vi "Scattered 2D Interpolation.vi"() -> ()   [LabVIEW 2023]
doc: "Illustrates how to use the Interpolate 2D Scattered VI to perform interpolation on scattered and grid data."
uses:
  <vilib>/Math Plots/3D Math Plots/3D Scatter/3D Scatter XCtrl/3D Scatter.xctl
  <vilib>/Math Plots/3D Math Plots/3D Surface/3D Surface XCtrl/3D Surface.xctl
  <vilib>/Analysis/1siggen.llb/Ramp Pattern by Samples.vi
  <vilib>/gmath/interp.llb/Create Mesh Grid (2D) (x,y arrays).vi
  <vilib>/Math Plots/3D Math Plots/3D Scatter/3D Scatter Datatype/Public/Plot Helper (Vector).vi
  <vilib>/gmath/interp.llb/Interpolate 2D Scattered (2D).vi
  <vilib>/Math Plots/3D Math Plots/3D Surface/3D Surface Datatype/Public/Plot Helper (Matrix).vi
  <vilib>/Analysis/NI_AALBase.lvlib
  <vilib>/gmath/NI_AAL_Interpolation.lvlib
  <vilib>/gmath/NI_Gmath.lvlib
  <vilib>/Math Plots/3D Math Plots/3D Scatter/3D Scatter Datatype/3D Scatter Datatype.lvclass
  <vilib>/Math Plots/3D Math Plots/3D Surface/3D Surface Datatype/3D Surface Datatype.lvclass
panel:
  out "Interpolation":refnum<class "3D Plot Datatype.lvclass">[](xcontrol)
  out "Raw Data":refnum<class "3D Plot Datatype.lvclass">[](xcontrol)
  in  "Data":u16(ring) items=["Scattered Data", "Grid Data"]
  in  "Method":i32(ring)=1 items=["nearest", "linear", "cubic", "biharmonic spline "]
  # "Overview: Illustrates how to use the Interpolate 2D Scattered VI to perform interpolation on scattered and grid data.\nRequirements: LabVIEW Full Development System\nInstructions: \n1. Use the Data option to choose between scattered or grid data.\n2. Use the Method option to choose the interpolation method.\n3. Run the VI.\n4. Observe the difference in input data types and interpolation methods on the Raw Data and Interpolation graphs."
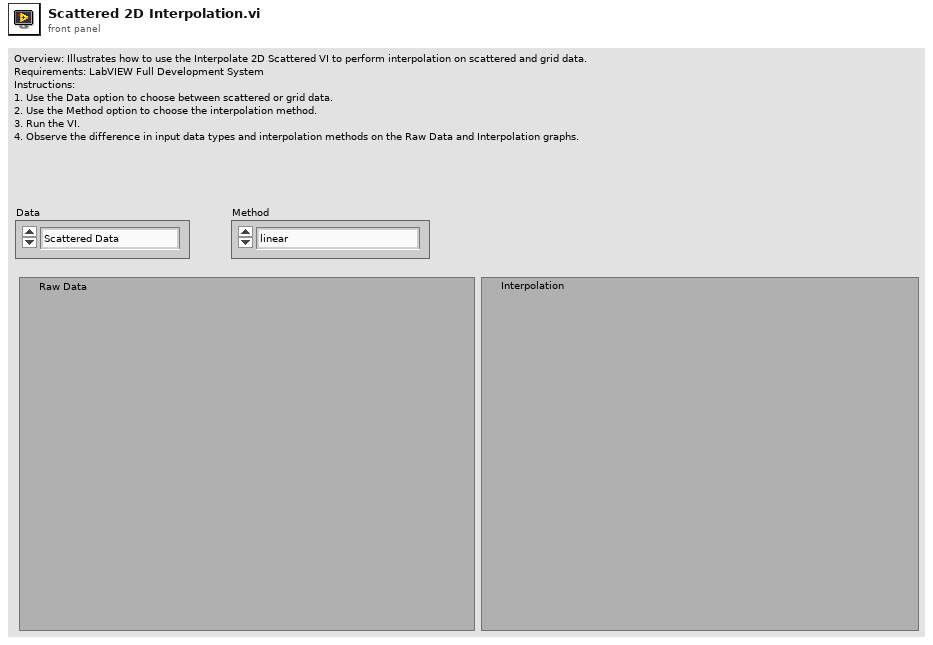
[diagram p1: front panel]
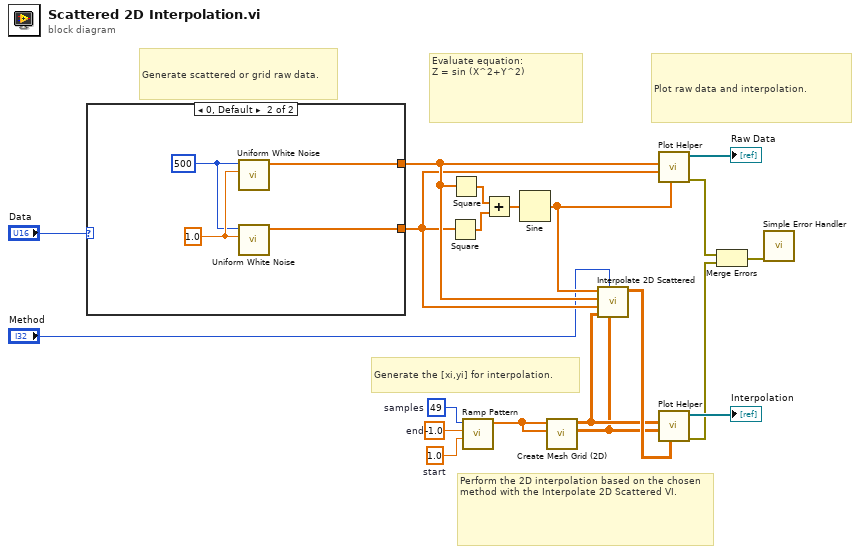
[diagram p0: block diagram]
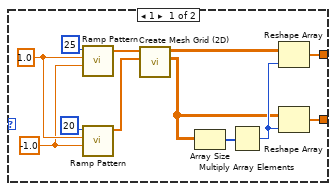
[diagram p2: hidden frame]
diagram:
  w13 = 1.0  # start
  w15 = 49  # samples
  w16 = -1.0  # end
  # "Generate the [xi,yi] for interpolation."
  # "Generate scattered or grid raw data."
  # "Perform the 2D interpolation based on the chosen method with the Interpolate 2D Scattered VI."
  # "Plot raw data and interpolation."
  # "Evaluate equation:\nZ = sin (X^2+Y^2)"
  n1 = case shown="0, Default" "Data" {
    tunnel: [w23 w33] -> w11
    tunnel: [w22 w34] -> w10
    frame 1 {
      w21 = -1.0 ("start")
      w31 = 1.0
      n2 = call-poly <vilib>:"Ramp Pattern.vi"("start"=w21, "end"=w31, "samples"=25) -> ("Ramp Pattern"=w30:dbl[])  [unwired: 7 in, 1 out]
      n3 = call-poly <vilib>:"Ramp Pattern.vi"("start"=w21, "end"=w31, "samples"=20) -> ("Ramp Pattern"=w29:dbl[])  [unwired: 7 in, 1 out]
      n4 = call-poly <vilib>:"Create Mesh Grid (2D).vi"("y domain"=w29, "x domain"=w30) -> ("Y"=w24:dbl[][], "X"=w27:dbl[][])  [unwired: 7 in, 1 out]
      n5 = Array Size(array=w24) -> (size(s)=w28:i32[])
      n6 = Multiply Array Elements(1:w28) -> (0:w26:i32)
      n7 = Reshape Array(w27, w26) -> (w23:dbl[])
      n8 = Reshape Array(w24, w26) -> (w22:dbl[])
    }
    frame 0, Default {
      w36 = 1.0
      w35 = 500 ("samples")
      n9 = call <vilib>:"Uniform White Noise.vi"("amplitude"=w36, "samples"=w35) -> ("uniform white noise"=w33:dbl[])  [unwired: 8 in, 1 out]
      n10 = call <vilib>:"Uniform White Noise.vi"("amplitude"=w36, "samples"=w35) -> ("uniform white noise"=w34:dbl[])  [unwired: 8 in, 1 out]
    }
  }
  n11 = Square(x=w10) -> (x^2=w20:dbl[])
  n12 = Square(x=w11) -> (x^2=w18:dbl[])
  n13 = call-poly <vilib>:"Ramp Pattern.vi"("start"=w13, "end"=w16, "samples"=w15) -> ("Ramp Pattern"=w14:dbl[])  [unwired: 7 in, 1 out]
  n14 = Add(x=w18, y=w20) -> (x+y=w19:dbl[])
  n15 = Sine(x=w19) -> (sin(x)=w9:dbl[])
  n16 = call-poly <vilib>:"Create Mesh Grid (2D).vi"("y domain"=w14, "x domain"=w14) -> ("Y"=w5:dbl[][], "X"=w6:dbl[][])  [unwired: 7 in, 1 out]
  n17 = call-poly <vilib>:"Interpolate 2D Scattered.vi"("Yi"=w5, "method"="Method", "Xi"=w6, "Y"=w10, "X"=w11, "Z"=w9) -> ("Zi"=w7:dbl[][])  [unwired: 4 in, 1 out]
  n18 = call-poly <vilib>:"Plot Helper.vi"("z vector"=w9, "y vector"=w10, "x vector"=w11) -> ("error out"=w4:errorcluster, "3D Plot lvclass Array out"=→"Raw Data":refnum<class "3D Plot Datatype.lvclass">[])  [unwired: 3 in, 4 out]
  n19 = call-poly <vilib>:"Plot Helper.vi"("z matrix"=w7, "y matrix"=w5, "x matrix"=w6) -> ("error out"=w3:errorcluster, "3D Plot lvclass Array out"=→"Interpolation":refnum<class "3D Plot Datatype.lvclass">[])  [unwired: 3 in, 4 out]
  n20 = Merge Errors(w4, w3) -> (w2:errorcluster)
  n21 = call <vilib>:"Simple Error Handler.vi"("error in (no error)"=w2) -> ()  [unwired: 4 in, 5 out]
